vi "Method One Return Value.vi"(8 "error in (no error)":errorcluster, 11 "Test Interface Mock in":refnum<class "Test Interface Mock.lvclass">) -> (0 "error out":errorcluster, 2 "Return Value":dbl, 3 "Test Interface Mock out":refnum<class "Test Interface Mock.lvclass">)   [LabVIEW 2020, in "Test Interface Mock.lvclass"]
uses:
  Test Interface Mock.lvclass
  C:/git/astemes-lmock/source/Framework/Mock/LMock Mock.lvclass
  source/Framework/Mock/LMock Mock.lvclass
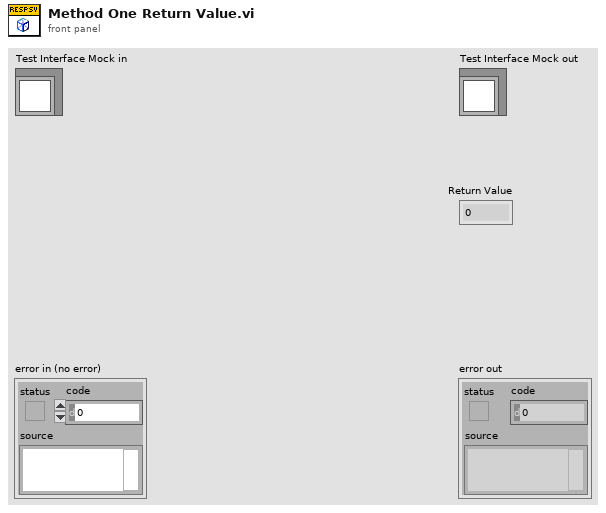
[diagram p1: front panel]
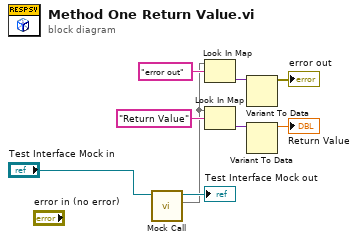
[diagram p0: block diagram]
diagram:
  n1 = call "Mock Call.vi"("Mock In"="Test Interface Mock in") -> ("Return Values"=w1:map{string, variant}, "Mock Out"=→"Test Interface Mock out":refnum<class "Test Interface Mock.lvclass">)  [unwired: 9 in]
  n2 = Look In Map(map=w1, key="error out") -> (value=w4:variant)  [unwired: 1 in, 1 out]
  n3 = Look In Map(map=w1, key="Return Value") -> (value=w6:variant)  [unwired: 1 in, 1 out]
  n4 = Variant To Data(Variant=w4) -> (data=→"error out":errorcluster)  [unwired: 2 in, 1 out]
  n5 = Variant To Data(Variant=w6) -> (data=→"Return Value":dbl)  [unwired: 2 in, 1 out]
